vi "Planner_Creator_Editor.vi"(8 "error in (no error)":errorcluster) -> (0 "error out":errorcluster)   [LabVIEW 2017]
uses:
  <vilib>/Utility/file.llb/Read Delimited Spreadsheet (string).vi
  <vilib>/Utility/file.llb/Write Delimited Spreadsheet (string).vi
  <vilib>/Utility/config.llb/NI_LVConfig.lvlib
panel:
  in  "BIN 2":T1
  in  "BIN 1":T1
  in  "SECTION No":string(combo)
  in  "Save Button":bool
  in  "HOME":bool
  in  "UPDATE TABLE":bool
  # "Plan Editor"
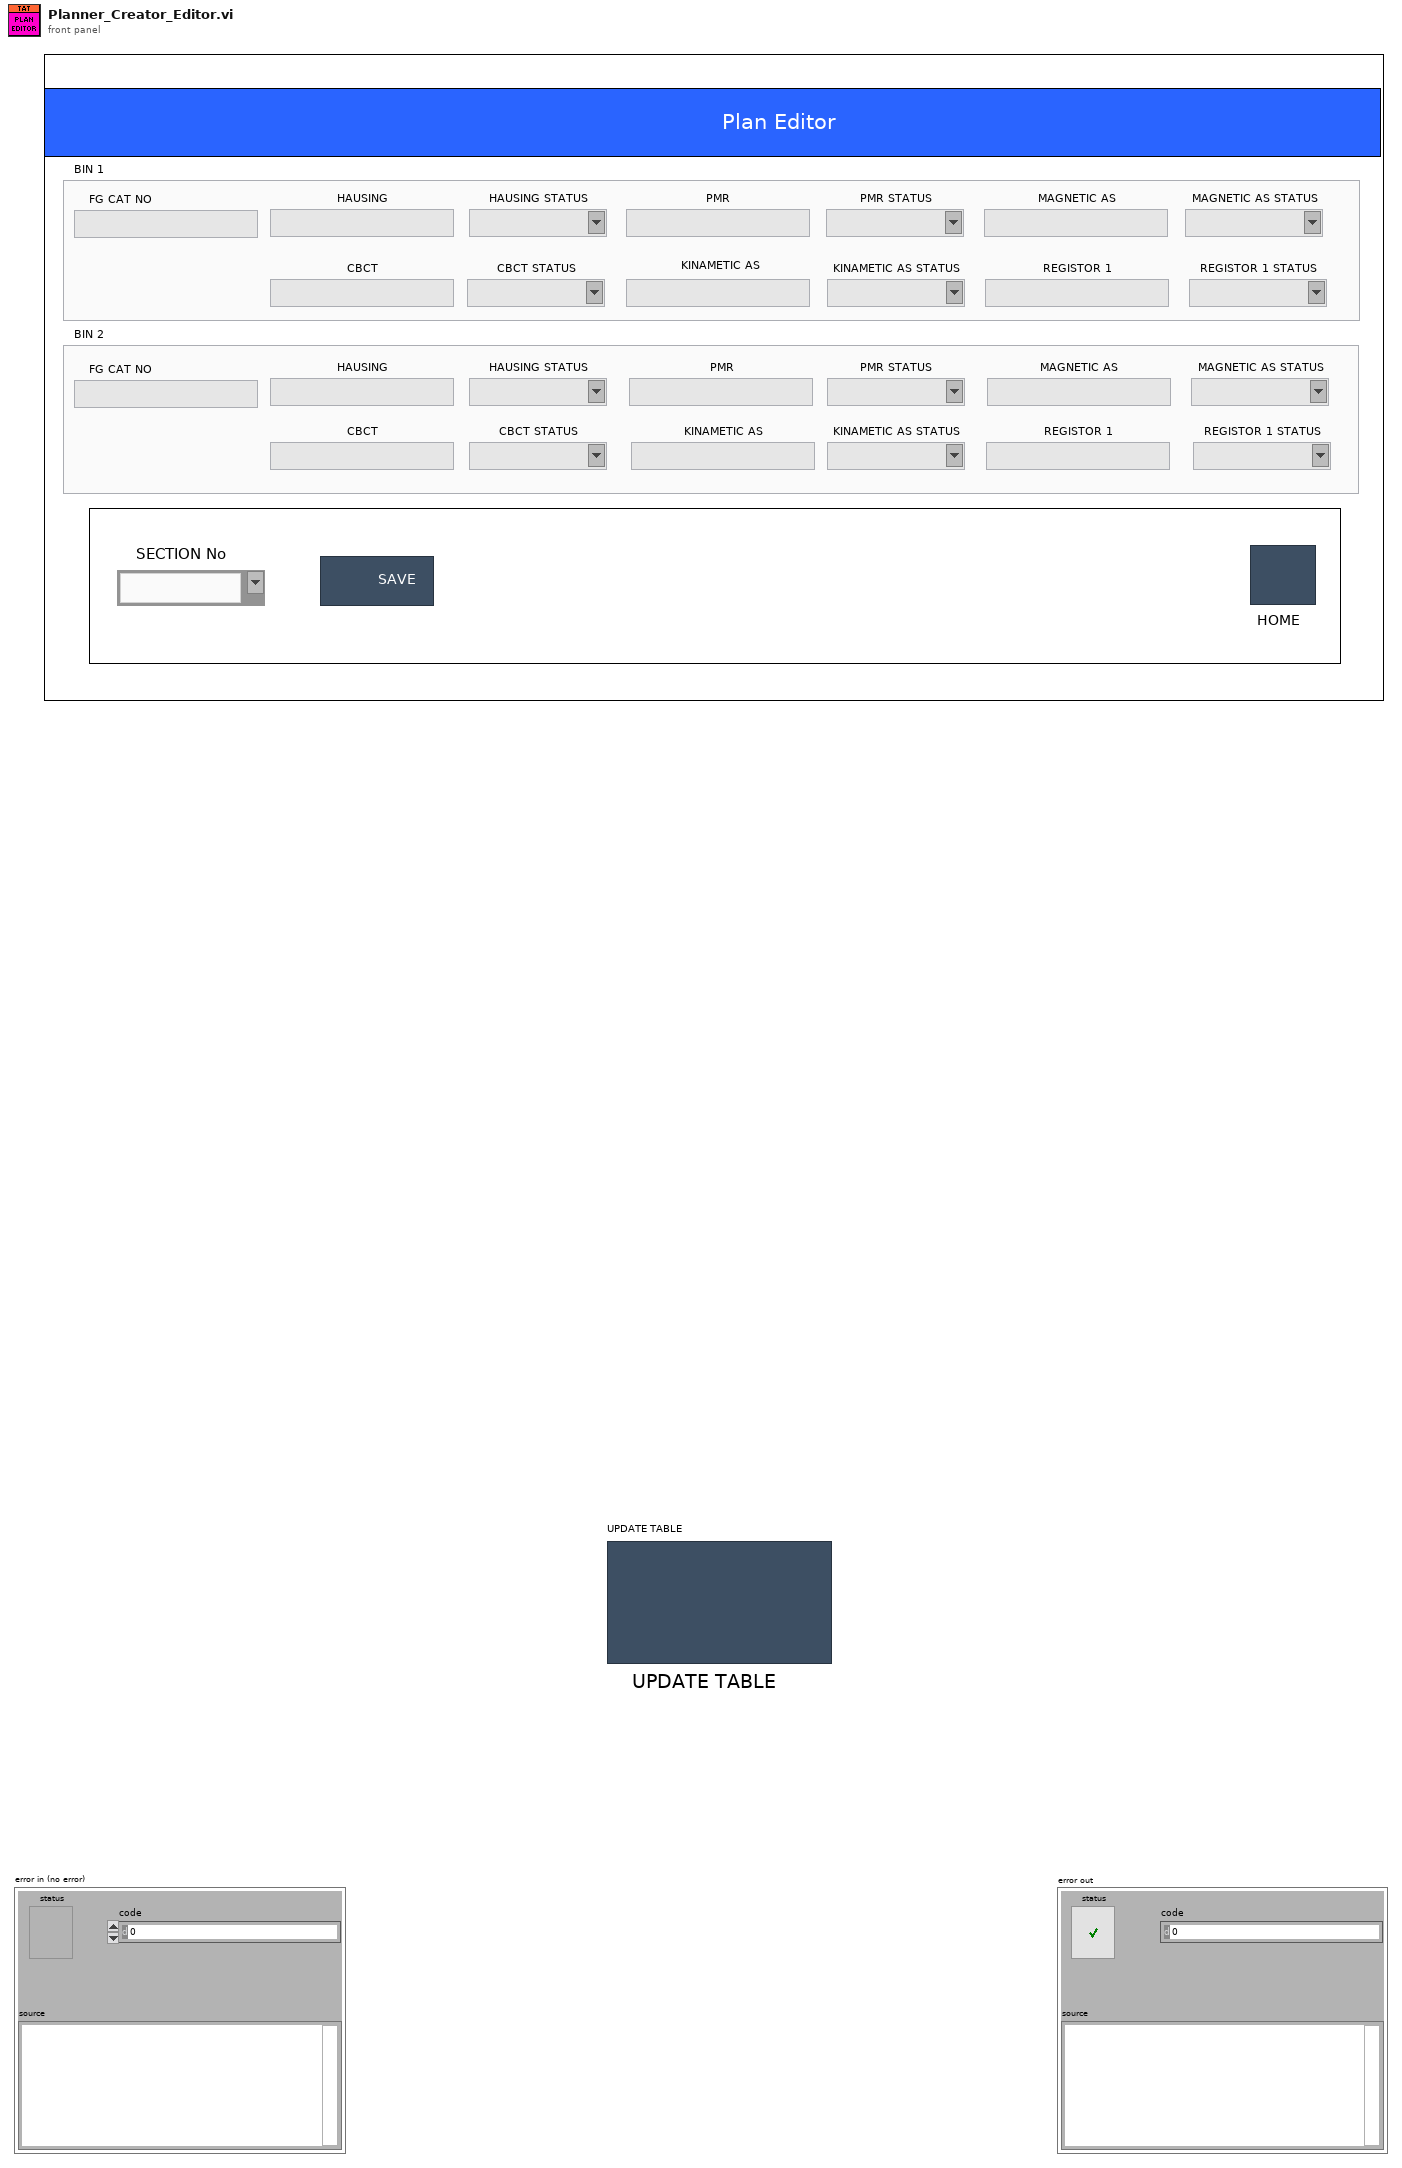
[diagram p1: front panel]
types:
  T1 = cluster{"FG CAT NO":string, "HAUSING":string, "HAUSING STATUS":string, "PMR":string, "PMR STATUS":string, "MAGNETIC AS":string, "MAGNETIC AS STATUS":string, "CBCT":string, "CBCT STATUS":string, "KINAMETIC AS":string, "KINAMETIC AS STATUS":string, "REGISTOR 1":string, "REGISTOR 1 STATUS":string}
  T2 = enum32{"invalid app kind", "Development System", "Run Time System", "Student Edition", "Embedded LabVIEW", "Evaluation", "Custom"}
  T3 = typedef "NI_LVConfig.lvlib/Config Data RefNum.ctl" = refnum<k1>
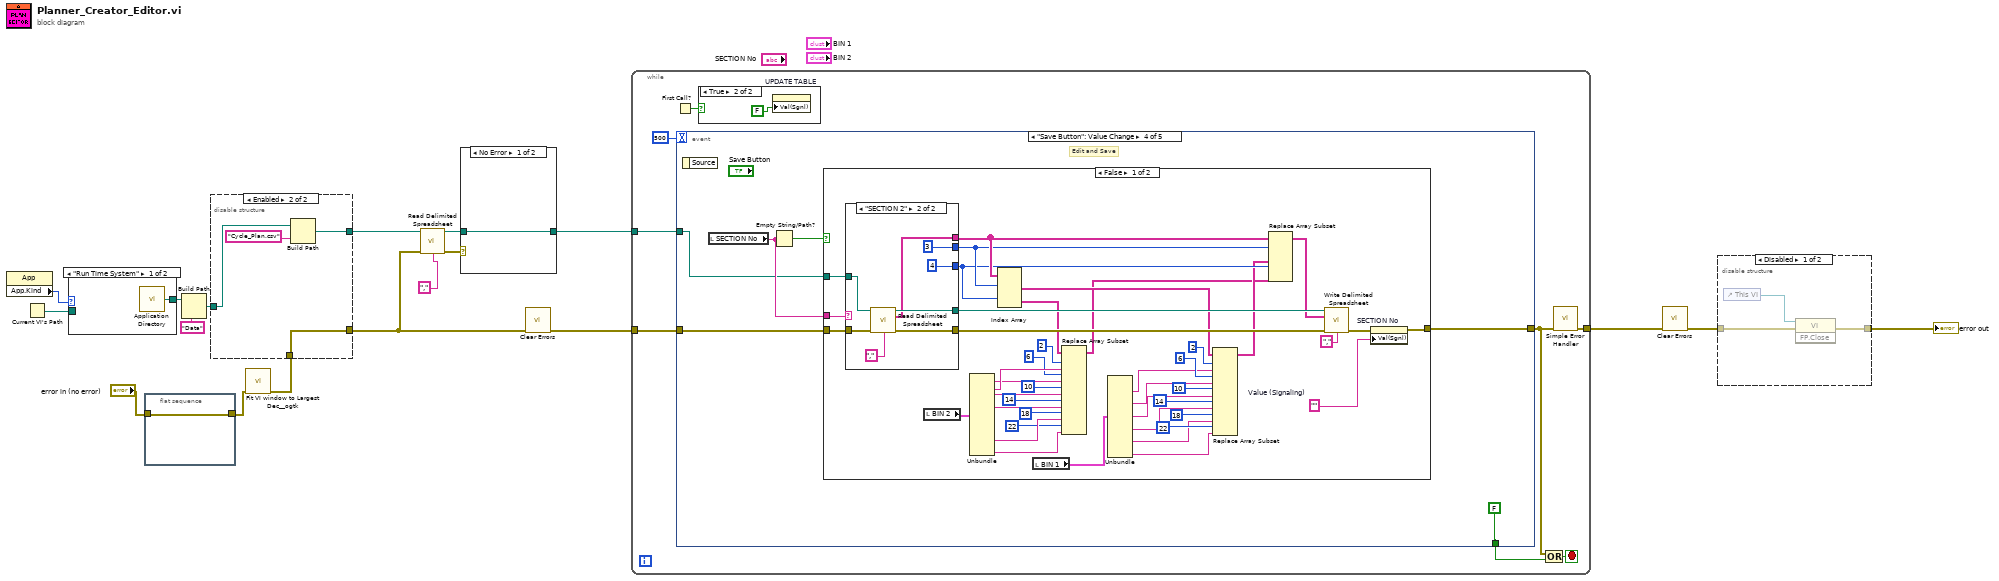
[diagram p0: block diagram]
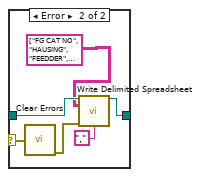
[diagram p2: hidden frame]
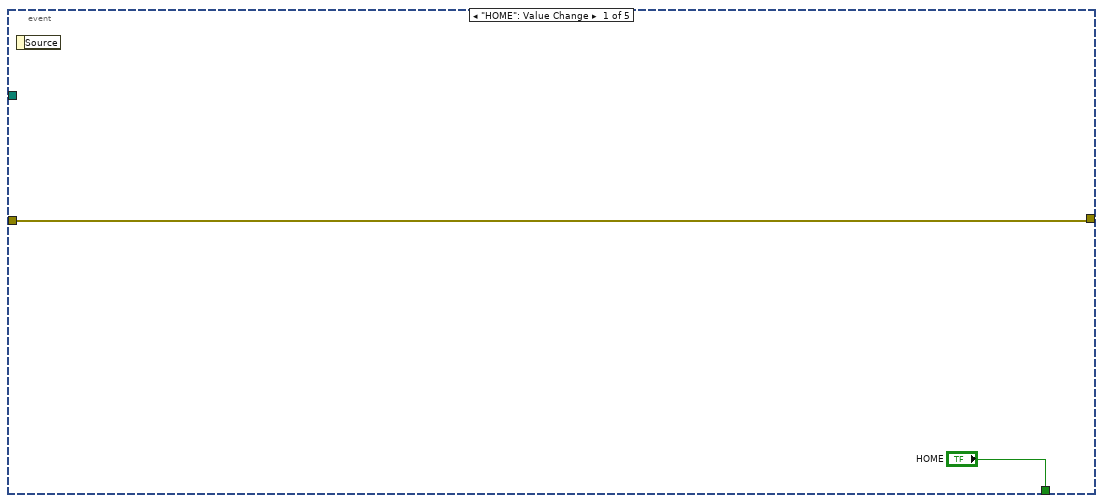
[diagram p4: hidden frame]
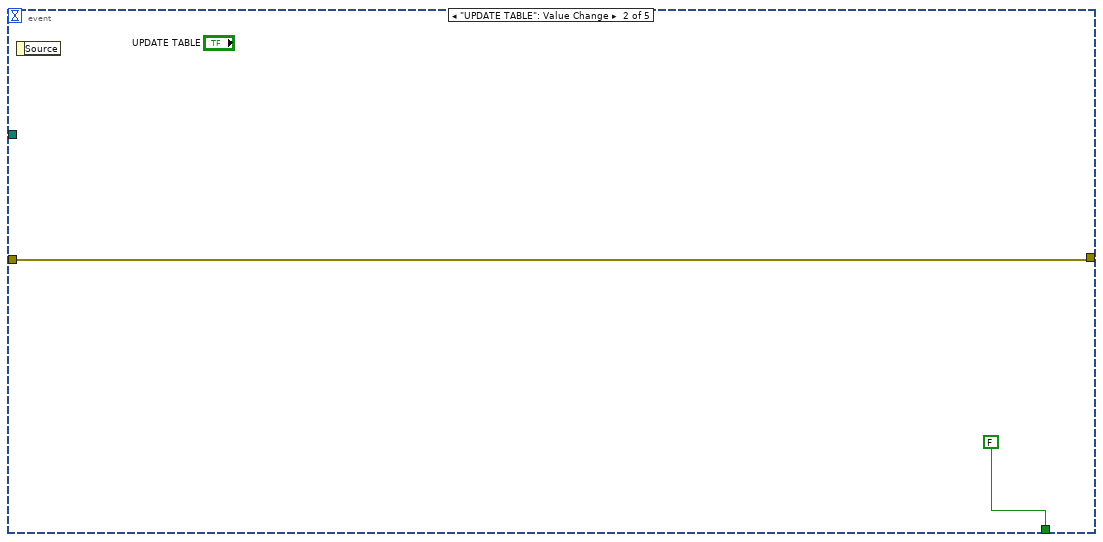
[diagram p5: hidden frame]
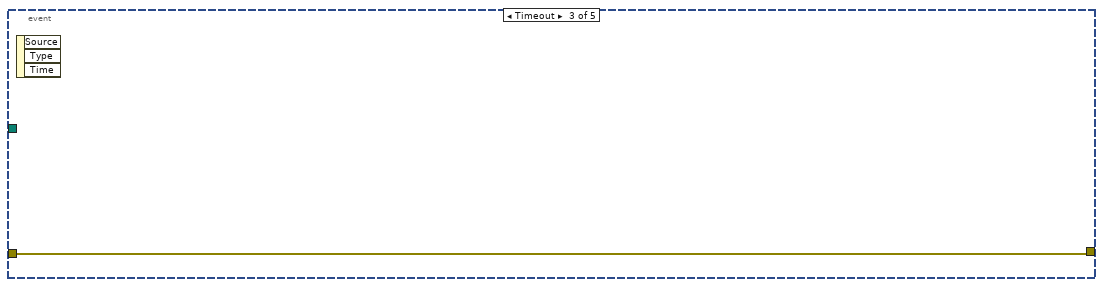
[diagram p6: hidden frame]
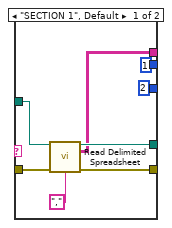
[diagram p7: hidden frame]
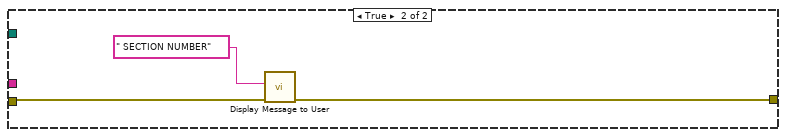
[diagram p8: hidden frame]
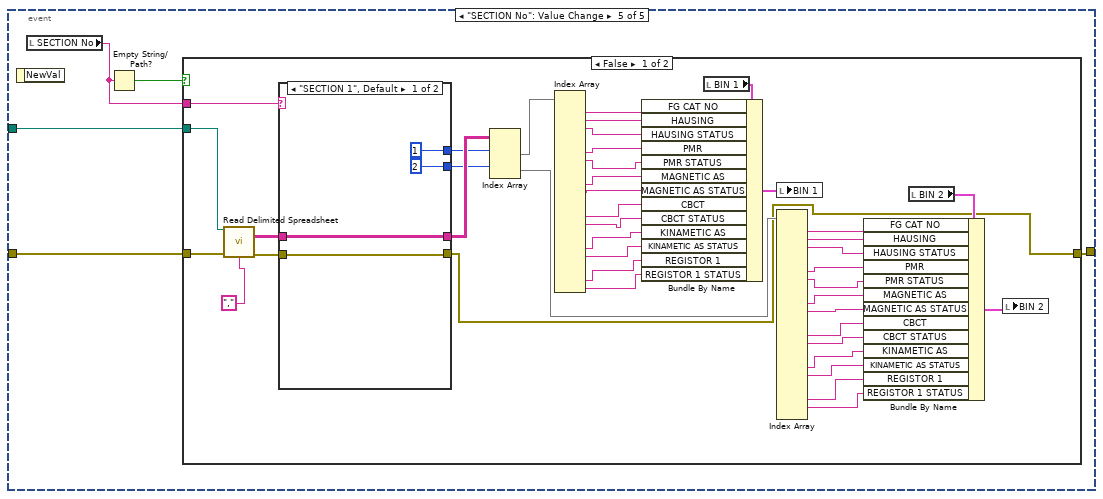
[diagram p9: hidden frame]
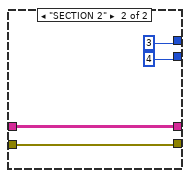
[diagram p10: hidden frame]
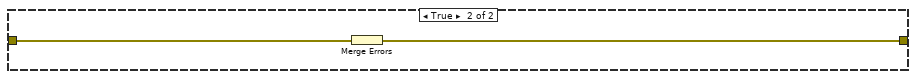
[diagram p11: hidden frame]
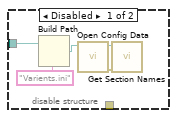
[diagram p13: hidden frame]
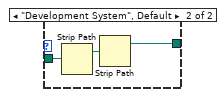
[diagram p14: hidden frame]
diagram:
  n1 = property class="App"() -> ("App.Kind"=w12:T2)  [unwired: 2 in, 2 out]
  n2 = Current VI's Path() -> (path=w13:path)
  n3 = case shown="\"Run Time System\"" w12 {
    tunnel: w13 -> [_ w21]
    tunnel: [w19 w20] -> w9
    frame "Run Time System" {
      n4 = call <vilib>:"Application Directory.vi"() -> ("Application Directory"=w19:path)
    }
    frame "Development System", Default {
      n5 = Strip Path(path=w21) -> (stripped path=w22:path)  [unwired: 1 out]
      n6 = Strip Path(path=w22) -> (stripped path=w20:path)  [unwired: 1 out]
    }
  }
  n7 = flat-sequence {
    tunnel: [w23] -> w14
    tunnel: "error in (no error)" -> [w23]
    frame #0 {
    }
  }
  n8 = Build Path(base path=w9, name or relative path="Data") -> (appended path=w10:path)
  n9 = call <userlib>:"Fit VI window to Largest Dec__ogtk.vi"("error in (no error)"=w14) -> ("error out"=w8:errorcluster)  [unwired: 5 in, 1 out]
  n10 = disable-structure shown="Enabled" {
    disable-tunnel: w10 -> [w24 w30]
    disable-tunnel: w8 -> [_ w32]
    disable-tunnel: [_ w32] -> w6
    disable-tunnel: [_ w29] -> w5
    frame Disabled {
      n11 = Build Path(base path=w24, name or relative path="Varients.ini") -> (appended path=w28:path)
      n12 = call <vilib>:"Open Config Data.vi"("configuration file path"=w28) -> ("error out"=w25:errorcluster, "refnum"=w26:T3)  [unwired: 8 in, 1 out]
      n13 = call <vilib>:"Get Section Names.vi"("error in (no error)"=w25, "refnum"=w26) -> ()  [unwired: 7 in, 3 out]
    }
    frame Enabled {
      n14 = Build Path(base path=w30, name or relative path="Cycle_Plan.csv") -> (appended path=w29:path)
    }
  }
  n15 = call-poly <vilib>:"Read Delimited Spreadsheet.vi"("file path (dialog if empty)"=w5, "error in (no error)"=w6, "delimiter (\\t)"=",") -> ("new file path (Not A Path if cancelled)"=w1:path, "error out"=w3:errorcluster)  [unwired: 7 in, 4 out]
  n16 = case shown="No Error" w3 {
    selector: w3 -> [_ w36]
    tunnel: [w33 w37] -> w2
    tunnel: w1 -> [w33 w38]
    frame No Error {
    }
    frame Error {
      n17 = call <vilib>:"Clear Errors.vi"("error in (no error)"=w36) -> ("error out"=w35:errorcluster)  [unwired: 5 in, 1 out]
      n18 = call-poly <vilib>:"Write Delimited Spreadsheet.vi"("file path (dialog if empty)"=w38, "2D data"=string[][] [["FG CAT NO", "HAUSING", "FEEDDER", "HAUSING_QR_CODE", "DOOR", "PMR", "FEEDDER", "PMR_QR_CODE", "DOOR", "MAGNETIC AS", "FEEDDER", "MAGNETIC AS_QR_CODE", "DOOR", "CBCT", "FEEDDER", "CBCT_QR_CODE", "DOOR", "KINAMETIC AS", "FEEDDER", "KINAMETIC AS_QR_CODE", "DOOR", "REGISTOR 1", "FEEDDER", "REGISTOR 1_QR_CODE", "DOOR", "QTY", "QTY_DONE"], ["Empty", "Empty", "Empty", "Empty", "Empty", "Empty", "Empty", "Empty", "Empty", "Empty", "Empty", "Empty", "Empty", "Empty", "Empty", "Empty", "Empty", "Empty", "Empty", "Empty", "Empty", "Empty", "Empty", "Empty", "Empty", "Empty", "Empty"], ["Empty", "Empty", "Empty", "Empty", "Empty", "Empty", "Empty", "Empty", "Empty", "Empty", "Empty", "Empty", "Empty", "Empty", "Empty", "Empty", "Empty", "Empty", "Empty", "Empty", "Empty", "Empty", "Empty", "Empty", "Empty", "Empty", "Empty"], ["Empty", "Empty", "Empty", "Empty", "Empty", "Empty", "Empty", "Empty", "Empty", "Empty", "Empty", "Empty", "Empty", "Empty", "Empty", "Empty", "Empty", "Empty", "Empty", "Empty", "Empty", "Empty", "Empty", "Empty", "Empty", "Empty", "Empty"], ["Empty", "Empty", "Empty", "Empty", "Empty", "Empty", "Empty", "Empty", "Empty", "Empty", "Empty", "Empty", "Empty", "Empty", "Empty", "Empty", "Empty", "Empty", "Empty", "Empty", "Empty", "Empty", "Empty", "Empty", "Empty", "Empty", "Empty"]], "error in (no error)"=w35, "delimiter (\\t)"=",") -> ("new file path (Not A Path if cancelled)"=w37:path)  [unwired: 10 in, 1 out]
    }
  }
  n19 = call <vilib>:"Clear Errors.vi"("error in (no error)"=w6) -> ("error out"=w7:errorcluster)  [unwired: 5 in, 1 out]
  n20 = while {
    tunnel: [w42] -> w16
    tunnel: w7 -> [w44]
    tunnel: w2 -> [w40]
    stop <- w46 stop-if-true
    n21 = First Call?() -> (First Call?: T/F=w45:bool)
    n22 = event shown="[3] \"Save Button\": Value Change" {
      selector: _ -> [_ _ _ _ _]
      dyn-events: _ -> [_ _ _ _ _]
      timeout: 500 -> [_ _ _ _ _]
      tunnel: ["HOME" FALSE ("stop") _ FALSE ("stop") _] -> w47
      tunnel: [w48 w50 w52 w57 w124] -> w43
      tunnel: w44 -> [w48 w50 w52 w56 w125]
      tunnel: w40 -> [_ _ _ w53 w121]
      event "HOME": Value Change {
        n23 = event-data() -> ()  [unwired: 1 in, 1 out]
      }
      event "UPDATE TABLE": Value Change {
        n24 = event-data() -> ()  [unwired: 1 in, 1 out]
      }
      event Timeout {
        n25 = event-data() -> ()  [unwired: 1 in, 3 out]
      }
      event "Save Button": Value Change {
        # "Edit and Save"
        n26 = event-data() -> ()  [unwired: 1 in, 1 out]
        n27 = local read "SECTION No"() -> (w54:string)
        n28 = Empty String/Path?(string/path=w54) -> (empty?=w55:bool)
        n29 = case shown="False" w55 {
          tunnel: [w101 w118] -> w57
          tunnel: w56 -> [w100 w119]
          tunnel: w54 -> [w99 _]
          tunnel: w53 -> [w98 _]
          frame False {
            w59 = ""  # Value (Signaling)
            n30 = case shown="\"SECTION 2\"" w99 {
              tunnel: w100 -> [w109 w117]
              tunnel: [w106 w116] -> w96
              tunnel: w98 -> [w107 w115]
              tunnel: [w105 w114] -> w97
              tunnel: [w104 w112] -> w91
              tunnel: [1 ("disabled index (col)") 3 ("disabled index (col)")] -> w90
              tunnel: [2 ("disabled index (col)") 4 ("disabled index (col)")] -> w89
              frame "SECTION 1", Default {
                n31 = call-poly <vilib>:"Read Delimited Spreadsheet.vi"("file path (dialog if empty)"=w107, "error in (no error)"=w109, "delimiter (\\t)"=",") -> ("new file path (Not A Path if cancelled)"=w105:path, "all rows"=w104:string[][], "error out"=w106:errorcluster)  [unwired: 7 in, 3 out]
              }
              frame "SECTION 2" {
                n32 = call-poly <vilib>:"Read Delimited Spreadsheet.vi"("file path (dialog if empty)"=w115, "error in (no error)"=w117, "delimiter (\\t)"=",") -> ("new file path (Not A Path if cancelled)"=w114:path, "all rows"=w112:string[][], "error out"=w116:errorcluster)  [unwired: 7 in, 3 out]
              }
            }
            n33 = local read "BIN 2"() -> (w92:T1)
            n34 = Unbundle(w92) -> ("HAUSING STATUS"=w87:string, "PMR STATUS"=w85:string, "MAGNETIC AS STATUS"=w83:string, "CBCT STATUS"=w81:string, "KINAMETIC AS STATUS"=w79:string, "REGISTOR 1 STATUS"=w77:string)  [unwired: 7 out]
            n35 = Index Array(array=w91, index (row) #1=w90, index (row) #2=w89) -> (element #1=w61:string[], element #2=w76:string[])  [unwired: 2 in]
            n36 = local read "BIN 1"() -> (w63:T1)
            n37 = Replace Array Subset(array=w76, new element #1=w87, index #1=2, new element #2=w85, index #2=6, new element #3=w83, index #3=10, new element #4=w81, index #4=14, new element #5=w79, index #5=18, new element #6=w77, index #6=22) -> (w60:string[])
            n38 = Unbundle(w63) -> ("HAUSING STATUS"=w65:string, "PMR STATUS"=w67:string, "MAGNETIC AS STATUS"=w69:string, "CBCT STATUS"=w71:string, "KINAMETIC AS STATUS"=w73:string, "REGISTOR 1 STATUS"=w75:string)  [unwired: 7 out]
            n39 = Replace Array Subset(array=w61, new element #1=w65, index #1=2, new element #2=w67, index #2=6, new element #3=w69, index #3=10, new element #4=w71, index #4=14, new element #5=w73, index #5=18, new element #6=w75, index #6=22) -> (w62:string[])
            n40 = Replace Array Subset(array=w91, new element #1=w62, index (row) #1=w90, new element #2=w60, index (row) #2=w89) -> (w93:string[][])  [unwired: 2 in]
            n41 = call-poly <vilib>:"Write Delimited Spreadsheet.vi"("file path (dialog if empty)"=w97, "2D data"=w93, "error in (no error)"=w96, "delimiter (\\t)"=",") -> ("error out"=w95:errorcluster)  [unwired: 10 in, 1 out]
            n42 = property on="SECTION No" class="CmbBox"(error in=w95, "Val(Sgnl)"=w59) -> (error out=w101:errorcluster)  [unwired: 1 in, 1 out]
          }
          frame True {
            n43 = call "Display Message to User"("error in (no error)"=w119, "Message"=" SECTION NUMBER") -> ("error out"=w118:errorcluster)  [unwired: 8 in, 1 out]
          }
        }
      }
      event "SECTION No": Value Change {
        n44 = event-data() -> ()  [unwired: 1 in, 1 out]
        n45 = local read "SECTION No"() -> (w123:string)
        n46 = Empty String/Path?(string/path=w123) -> (empty?=w122:bool)
        n47 = case shown="False" w122 {
          tunnel: w125 -> [w163 w177]
          tunnel: [w138 w176] -> w124
          tunnel: w123 -> [w167 _]
          tunnel: w121 -> [w162 _]
          frame False {
            n48 = call-poly <vilib>:"Read Delimited Spreadsheet.vi"("file path (dialog if empty)"=w162, "error in (no error)"=w163, "delimiter (\\t)"=",") -> ("all rows"=w160:string[][], "error out"=w161:errorcluster)  [unwired: 7 in, 4 out]
            n49 = case shown="\"SECTION 1\", Default" w167 {
              tunnel: [w171 w175] -> w138
              tunnel: w161 -> [w171 w175]
              tunnel: w160 -> [w170 w172]
              tunnel: [w170 w172] -> w159
              tunnel: [1 3] -> w158
              tunnel: [2 4] -> w157
              frame "SECTION 1", Default {
              }
              frame "SECTION 2" {
              }
            }
            n50 = Index Array(array=w159, index (row) #1=w158, index (row) #2=w157) -> (element #1=w156:string[], element #2=w141:string[])  [unwired: 2 in]
            n51 = Index Array(array=w156) -> (element #1=w155:string, element #2=w154:string, element #3=w137:string, element #6=w153:string, element #7=w136:string, element #10=w152:string, element #11=w135:string, element #14=w151:string, element #15=w134:string, element #18=w150:string, element #19=w133:string, element #22=w149:string, element #23=w132:string)  [unwired: 23 in, 10 out]
            n52 = local read "BIN 1"() -> (w165:T1)
            n53 = Bundle By Name(cluster=w165, "FG CAT NO"=w155, "HAUSING"=w154, "HAUSING STATUS"=w137, "PMR"=w153, "PMR STATUS"=w136, "MAGNETIC AS"=w152, "MAGNETIC AS STATUS"=w135, "CBCT"=w151, "CBCT STATUS"=w134, "KINAMETIC AS"=w150, "KINAMETIC AS STATUS"=w133, "REGISTOR 1"=w149, "REGISTOR 1 STATUS"=w132) -> (w166:T1)
            n54 = local write "BIN 1"(w166) -> ()
            n55 = Index Array(array=w141) -> (element #1=w142:string, element #2=w143:string, element #3=w131:string, element #6=w144:string, element #7=w130:string, element #10=w145:string, element #11=w129:string, element #14=w146:string, element #15=w128:string, element #18=w147:string, element #19=w127:string, element #22=w148:string, element #23=w126:string)  [unwired: 24 in, 11 out]
            n56 = local read "BIN 2"() -> (w140:T1)
            n57 = Bundle By Name(cluster=w140, "FG CAT NO"=w142, "HAUSING"=w143, "HAUSING STATUS"=w131, "PMR"=w144, "PMR STATUS"=w130, "MAGNETIC AS"=w145, "MAGNETIC AS STATUS"=w129, "CBCT"=w146, "CBCT STATUS"=w128, "KINAMETIC AS"=w147, "KINAMETIC AS STATUS"=w127, "REGISTOR 1"=w148, "REGISTOR 1 STATUS"=w126) -> (w139:T1)
            n58 = local write "BIN 2"(w139) -> ()
          }
          frame True {
            n59 = Merge Errors(w177) -> (w176:errorcluster)
          }
        }
      }
    }
    n60 = case shown="True" w45 {
      frame False {
      }
      frame True {
        n61 = property on="UPDATE TABLE" class="Bool (strict)"("Val(Sgnl)"=FALSE) -> ()  [unwired: 2 in, 2 out]
      }
    }
    n62 = Or(x=w43, y=w47) -> (x .or. y?=w46:bool)
    n63 = call <vilib>:"Simple Error Handler.vi"("error in (no error)"=w43) -> ("error out"=w42:errorcluster)  [unwired: 4 in, 4 out]
  }
  n64 = call <vilib>:"Clear Errors.vi"("error in (no error)"=w16) -> ("error out"=w18:errorcluster)  [unwired: 5 in, 1 out]
  n65 = disable-structure shown="Disabled" {
    disable-tunnel: w18 -> [w181 w182]
    disable-tunnel: [w180 w182] -> w17
    frame Disabled {
      n66 = control-ref of="This VI"() -> (w179:refnum<vi>)
      n67 = invoke class="VI" method="FP.Close"(reference=w179, error in=w181) -> (error out=w180:errorcluster)  [unwired: 1 in, 2 out]
    }
    frame Enabled {
    }
  }
  "error out" <- w17
